vi "ReadB.vi"(8 "error in (no error)":errorcluster, 10 "Offset":u32) -> (0 "error out":errorcluster, 2 "Data 2":u8=255, 3 "Data 1":u8=255)   [LabVIEW 2015, in "ESLSCDLL.lvlib"]
uses:
  ESLSCDLL.lvlib
  Globals.vi
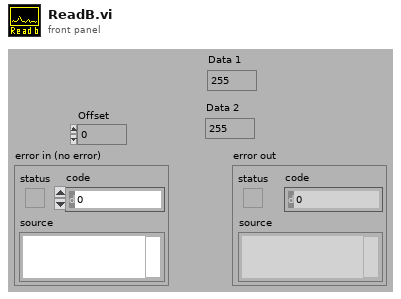
[diagram p1: front panel]
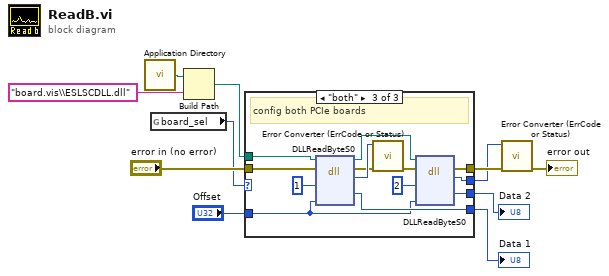
[diagram p0: block diagram]
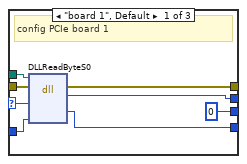
[diagram p2: hidden frame]
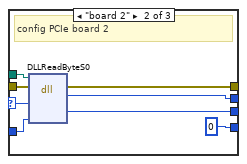
[diagram p3: hidden frame]
diagram:
  n1 = call <vilib>:"Application Directory.vi"() -> ("Application Directory"=w3:path)
  n2 = global read "Globals.vi" "board_sel"() -> (w4:enum32{"0", "board 1", "board 2", "both"})
  n3 = Build Path(base path=w3, name or relative path="board.vis\\ESLSCDLL.dll") -> (appended path=w1:path)
  n4 = case shown="\"both\"" w4 {
    selector: w4 -> [w17 w27 _]
    tunnel: [w19 u8 0 w40] -> w11
    tunnel: "Offset" -> [w18 w26 w36]
    tunnel: [u8 0 w25 w39] -> w9
    tunnel: "error in (no error)" -> [w15 w23 w33]
    tunnel: [w14 w22 w31] -> w6
    tunnel: [w13 w21 w30] -> w5
    tunnel: w1 -> [w12 w20 w29]
    frame "board 1", Default {
      # "config PCIe board 1"
      n5 = dll-call lib="C:/ENTW/PCIE/LV64/board.vis/ESLSCDLL.dll" fn="DLLReadByteS0"(path in=w12, error in=w15, "drv"=w17, "PortOff"=w18) -> (error out=w14:errorcluster, "es_status_codes"=w13:i32, "data"=w19:u8)  [unwired: 4 in, 1 out]
    }
    frame "board 2" {
      # "config PCIe board 2"
      n6 = dll-call lib="C:/ENTW/PCIE/LV64/board.vis/ESLSCDLL.dll" fn="DLLReadByteS0"(path in=w20, error in=w23, "drv"=w27, "PortOff"=w26) -> (error out=w22:errorcluster, "es_status_codes"=w21:i32, "data"=w25:u8)  [unwired: 4 in, 1 out]
    }
    frame "both" {
      # "config both PCIe boards"
      n7 = dll-call lib="C:/ENTW/PCIE/LV64/board.vis/ESLSCDLL.dll" fn="DLLReadByteS0"(path in=w29, error in=w33, "drv"=u32 1, "PortOff"=w36) -> (path out=w28:path, error out=w34:errorcluster, "es_status_codes"=w35:i32, "data"=w40:u8)  [unwired: 4 in]
      n8 = call "Error Converter (ErrCode or Status).vi"("error in (no error)"=w34, "error code"=w35) -> ("error out"=w32:errorcluster)  [unwired: 9 in]
      n9 = dll-call lib="C:/ENTW/PCIE/LV64/board.vis/ESLSCDLL.dll" fn="DLLReadByteS0"(path in=w28, error in=w32, "drv"=u32 2, "PortOff"=w36) -> (error out=w31:errorcluster, "es_status_codes"=w30:i32, "data"=w39:u8)  [unwired: 4 in, 1 out]
    }
  }
  "Data 1" <- w11
  "Data 2" <- w9
  n10 = call "Error Converter (ErrCode or Status).vi"("error in (no error)"=w6, "error code"=w5) -> ("error out"=→"error out":errorcluster)  [unwired: 9 in]
